vi "Observe Data.vi"(6 "Time Stamp":timestamp, 8 "error in (no error)":errorcluster, 9 "Value":variant, 10 "Datum Name":string, 11 "IObserver in":refnum<class "IObserver.lvclass">) -> (0 "error out":errorcluster, 3 "IObserver out":refnum<class "IObserver.lvclass">)   [LabVIEW 2019, in "IObserver.lvlib" / "IObserver.lvclass"]
doc: "<License>\nCopyright © 2017 Composed Systems, LLC | All rights reserved\nwww.composed.io\n\nAuthor: Ethan Stern <ethan.stern@composed.io>\n\nThis software is provided \"AS IS\" WITHOUT WARRANTIES, either express or implied, AND IS FOR EDUCATIONAL PURPOSES ONLY.\n</License>"
uses:
  <vilib>/gpm_packages/@cs/mva-core/Source/IObserver/IObserver/IObserver.lvclass
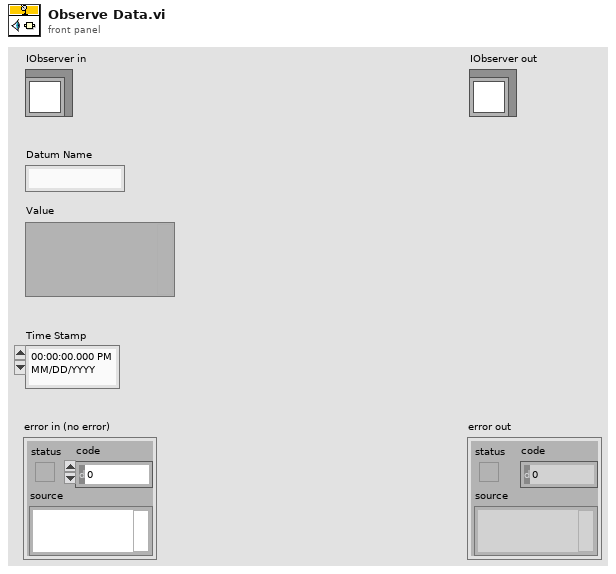
[diagram p1: front panel]
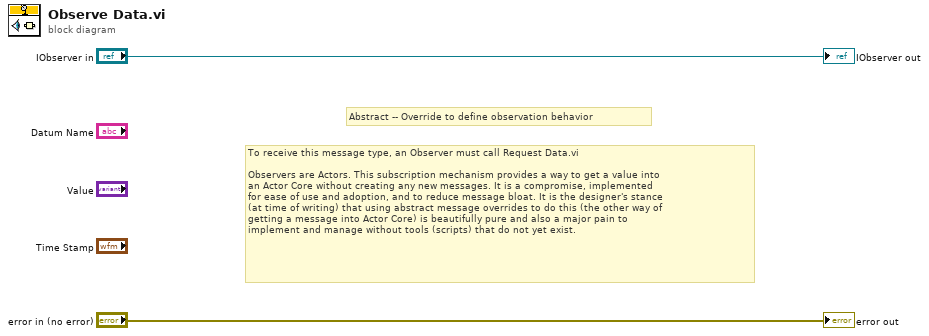
[diagram p0: block diagram]
diagram:
  # "To receive this message type, an Observer must call Request Data.vi\n\nObservers are Actors. This subscription mechanism provides a way to get a value into\nan Actor Core without creating any new messages. It is a compromise, implemented\nfor ease of use and adoption, and to reduce message bloat. It is the designer's stance\n(at time of writing) that using abstract message overrides to do this (the other way of\ngetting a message into Actor Core) is beautifully pure and also a major pain to\nimplement and manage without tools (scripts) that do not yet exist."
  # "Abstract -- Override to define observation behavior"
  "error out" <- "error in (no error)"
  "IObserver out" <- "IObserver in"
